vi "Configure Receiver Leveling Sweep.vi"(0 "VISA resource name":refnum<visa-resource-name>, 1 "Channel (1)":i32=1, 2 "Port ( 1)":i32=1, 3 "Enable Fast IF Bandwidth (F: Disabled)":bool, 4 "IF Bandwidth (70000)":dbl=70000.0, 5 "error in (no error)":errorcluster, 6 "Enable Receiver Leveling (F: Disabled)":bool, 7 "Power Level Offset (0)":dbl, 8 "Maximum Iterations to Tolerance (5)":dbl=5.0, 9 "Tolerance Level (5)":dbl=5.0, 10 "Reference Receiver (0: R1)":i32(ring) items=["R1", "R2", "A", "B"]) -> (14 "VISA resource name out":refnum<visa-resource-name>, 19 "error out":errorcluster)   [LabVIEW 2020, in "Agilent ENA Series.lvlib"]
doc: "Configures numerous settings related to the receiver leveling sweep. \n\nNote:\nValid for E5072A only."
uses:
  <instrlib>/Agilent ENA Series/Agilent ENA Series.lvlib
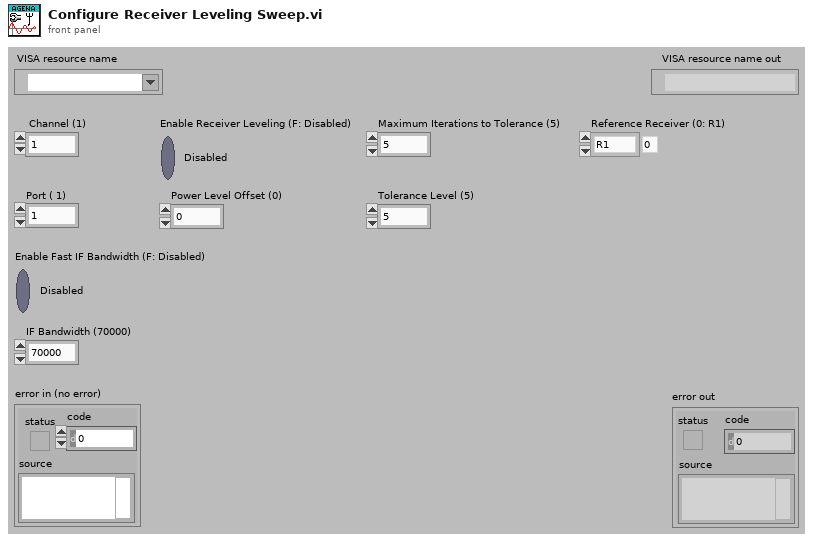
[diagram p1: front panel]
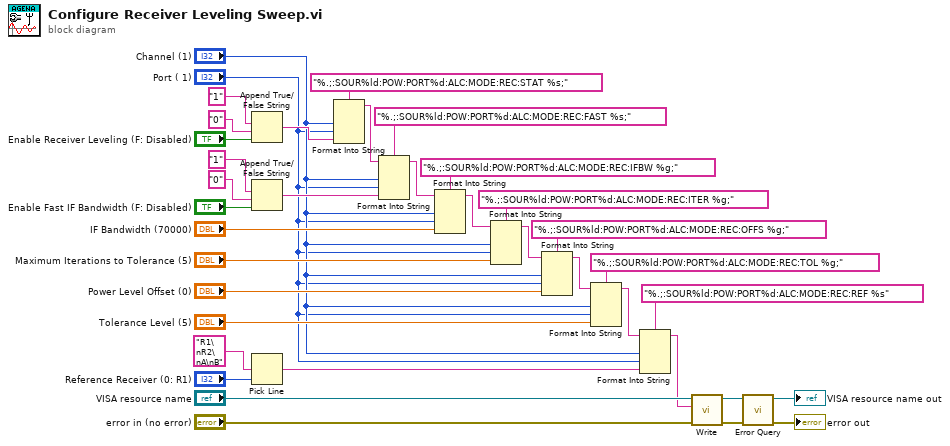
[diagram p0: block diagram]
diagram:
  n1 = Append True/False String(1:"Enable Receiver Leveling (F: Disabled)", 2:"0" ("false string"), 3:"1" ("true string")) -> (0:w27:string)  [unwired: 1 in]
  n2 = Append True/False String(1:"Enable Fast IF Bandwidth (F: Disabled)", 2:"0" ("false string"), 3:"1" ("true string")) -> (0:w23:string)  [unwired: 1 in]
  n3 = Pick Line(multi-line string="R1\nR2\nA\nB", line index="Reference Receiver (0: R1)") -> (output string=w7:string)  [unwired: 1 in]
  n4 = Format Into String(format string="%.;:SOUR%ld:POW:PORT%d:ALC:MODE:REC:STAT %s;", "Channel (1)", "Port ( 1)", w27) -> (resulting string=w22:string)  [unwired: 2 in, 1 out]
  n5 = Format Into String(format string="%.;:SOUR%ld:POW:PORT%d:ALC:MODE:REC:FAST %s;", initial string=w22, "Channel (1)", "Port ( 1)", w23) -> (resulting string=w19:string)  [unwired: 1 in, 1 out]
  n6 = Format Into String(format string="%.;:SOUR%ld:POW:PORT%d:ALC:MODE:REC:IFBW %g;", initial string=w19, "Channel (1)", "Port ( 1)", "IF Bandwidth (70000)") -> (resulting string=w4:string)  [unwired: 1 in, 1 out]
  n7 = Format Into String(format string="%.;:SOUR%ld:POW:PORT%d:ALC:MODE:REC:ITER %g;", initial string=w4, "Channel (1)", "Port ( 1)", "Maximum Iterations to Tolerance (5)") -> (resulting string=w3:string)  [unwired: 1 in, 1 out]
  n8 = Format Into String(format string="%.;:SOUR%ld:POW:PORT%d:ALC:MODE:REC:OFFS %g;", initial string=w3, "Channel (1)", "Port ( 1)", "Power Level Offset (0)") -> (resulting string=w2:string)  [unwired: 1 in, 1 out]
  n9 = Format Into String(format string="%.;:SOUR%ld:POW:PORT%d:ALC:MODE:REC:TOL %g;", initial string=w2, "Channel (1)", "Port ( 1)", "Tolerance Level (5)") -> (resulting string=w11:string)  [unwired: 1 in, 1 out]
  n10 = Format Into String(format string="%.;:SOUR%ld:POW:PORT%d:ALC:MODE:REC:REF %s", initial string=w11, "Channel (1)", "Port ( 1)", w7) -> (resulting string=w1:string)  [unwired: 1 in, 1 out]
  n11 = call <instrlib>:"Write.vi"("error in (no error)"="error in (no error)", "String ()"=w1, "VISA resource name"="VISA resource name") -> ("error out"=w34:errorcluster, "VISA resource name out"=w35:refnum<visa-resource-name>)  [unwired: 6 in, 1 out]
  n12 = call <instrlib>:"Error Query.vi"("error in (no error)"=w34, "VISA resource name"=w35) -> ("error out"=→"error out":errorcluster, "VISA resource name out"=→"VISA resource name out":refnum<visa-resource-name>)  [unwired: 6 in, 2 out]
